vi "Serialize.vi"(8 "error in":errorcluster, 9 "OwningElement in":refnum<k20>, 10 "Document in":refnum<k20>, 11 "Attribute in":refnum<class "Attribute.lvclass">) -> (0 "error out":errorcluster, 1 "OwningElement out":refnum<k20>, 2 "Document out":refnum<k20>, 3 "Attribute out":refnum<class "Attribute.lvclass">)   [LabVIEW 2021, in "ProligentXMLGenerator.lvlib" / "Attribute.lvclass"]
uses:
  Attribute.lvclass
  Attribute.lvclass/Attribute.ctl
  DOMSupport/DOMSupport.lvlib
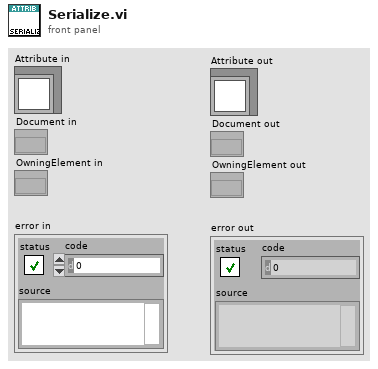
[diagram p1: front panel]
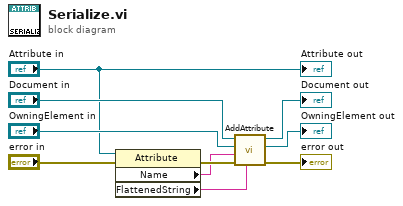
[diagram p0: block diagram]
diagram:
  n1 = property on="Property Node" class="Attribute"(reference="Attribute in", error in="error in") -> (error out=w10:errorcluster, "Name"=w9:string, "FlattenedString"=w4:string)  [unwired: 1 out]
  n2 = call "AddAttribute.vi"("Value"=w4, "error in"=w10, "Name"=w9, "OwningElement in"="OwningElement in", "Document in"="Document in") -> ("error out"=→"error out":errorcluster, "OwningElement out"=→"OwningElement out":refnum<k20>, "Document out"=→"Document out":refnum<k20>)  [unwired: 4 in]
  "Attribute out" <- "Attribute in"
